vi "ScanFSM.vi"(0 "FSM X Task":refnum<k21>, 1 "FSM Y Task":refnum<k21>, 3 "Scan XY Map Progess Bar":refnum<vi>, 4 "XY Map Expected (s)":refnum<vi>, 5 "XY Map Elapsed (s)":refnum<vi>, 6 "XY Intensity Map":refnum<vi>, 7 "Scan X Readout (V)":refnum<vi>, 8 "CCD 1D Spectrum XY Map":refnum<vi>, 9 "LightField Automation out":refnum<class "LightField Automation.lvclass">, 10 "Params XY Map SubVI":T4, 11 "Scan Y Readout (V)":refnum<vi>, 12 "Scan XY Map Exp Params SubVI":T3, 13 "Stop XY Map":refnum<vi>, 14 "CCD 2D Image XY Map":refnum<vi>, 19 "LightField Automation error out":errorcluster) -> (16 "Data":i32[][](array[numeric]), 17 "LF Out":refnum<class "LightField Automation.lvclass">, 18 "LF Error Out":errorcluster)   [LabVIEW 2019]
uses:
  TypeDefs/AcqMode.ctl
  Light Field/lightfield-automation-labview/LightField Automation.lvclass
panel:
  out "size(s)":i32[](array[numeric])
  out "Numeric 2":i32
  out "Numeric":i32
  out "Number of points":dbl=121.0
  out "YMultiplier":dbl
  out "YOffset":dbl
  out "XMultiplier":dbl
  out "XOffset":dbl
  out "XYPos Indices Randomized":dbl[][](array[numeric])
  out "XYPos Indices":i32[][](array[numeric])
  out "Random index":i32[](array[numeric])=[4, 16, 17, 14, 92, 29, 8, 31, 42, 104, 84, 28, 85, 90, 13, 60, 120, 41, 111, 82, 69, 34, 7, 77, 47, 59, 65, 116, 24, 30, 113, 2, 63, 94, 106, 103, 71, 100, 22, 18, 32, 102, 19, 97, 44, 12, 0, 1, 109, 27, 88, 99, 51, 107, 76, 56, 81, 96, 72, 93, 74, 21, 5, 79, 9, 117, 38, 45, 25, 58, 105, 57, 40, 52, 23, 87, 89, 62, 26, 110, 37, 3, 101, 10, 54, 61, 83, 46, 86, 66, 68, 43, 108, 11, 67, 75, 6, 80, 49, 20, 112, 78, 115, 119, 95, 64, 73, 39, 15, 48, 55, 70, 50, 98, 91, 35, 53, 36, 118, 33, 114]
  out "X size":dbl=11.0
  out "Y size":dbl=11.0
  out "WL Calib":dbl[](array[numeric])
  out "CCD 1D Spectrum XY Map 2":cluster{dbl[], dbl[]}(graph)
  out "CCD ROI":T1(ring)
  out "Accumulations":dbl
  out "Acq Mode":T2=enum."Spectrum"
  out "KCube Shutter On?":bool
  out "A Time (ms)":dbl
  out "XY Intensity Map":dbl[][](graph)=[[3.904687043201515e-13, 6.684989195773002e-11, 3.649880430807626e-09, 6.355065252727497e-08, 3.5287820878809013e-07, 6.248749509463085e-07, 3.5287820878809013e-07, 6.355065252727497e-08, 3.649880430807626e-09, 6.684989195773002e-11, 3.904687043201515e-13], [6.684989195773002e-11, 1.1444983952148092e-08, 6.248749509463097e-07, 1.0880140221963334e-05, 6.041424029819161e-05, 0.0001069812317752422, 6.041424029819161e-05, 1.0880140221963334e-05, 6.248749509463097e-07, 1.1444983952148092e-08, 6.684989195773002e-11], [3.649880430807626e-09, 6.248749509463097e-07, 3.41170163237202e-05, 0.0005940355282204004, 0.003298505755939091, 0.005840977343195246, 0.003298505755939091, 0.0005940355282204004, 3.41170163237202e-05, 6.248749509463097e-07, 3.649880430807626e-09], [6.355065252727497e-08, 1.0880140221963334e-05, 0.0005940355282204004, 0.01034317319661825, 0.05743261926761737, 0.10170139230422684, 0.05743261926761737, 0.01034317319661825, 0.0005940355282204004, 1.0880140221963334e-05, 6.355065252727497e-08], [3.5287820878809013e-07, 6.041424029819161e-05, 0.003298505755939091, 0.05743261926761737, 0.31890655732397044, 0.5647181220077593, 0.31890655732397044, 0.05743261926761737, 0.003298505755939091, 6.041424029819161e-05, 3.5287820878809013e-07], [6.248749509463085e-07, 0.0001069812317752422, 0.005840977343195246, 0.10170139230422684, 0.5647181220077593, 1.0, 0.5647181220077593, 0.10170139230422684, 0.005840977343195246, 0.0001069812317752422, 6.248749509463085e-07], [3.5287820878809013e-07, 6.041424029819161e-05, 0.003298505755939091, 0.05743261926761737, 0.31890655732397044, 0.5647181220077593, 0.31890655732397044, 0.05743261926761737, 0.003298505755939091, 6.041424029819161e-05, 3.5287820878809013e-07], [6.355065252727497e-08, 1.0880140221963334e-05, 0.0005940355282204004, 0.01034317319661825, 0.05743261926761737, 0.10170139230422684, 0.05743261926761737, 0.01034317319661825, 0.0005940355282204004, 1.0880140221963334e-05, 6.355065252727497e-08], [3.649880430807626e-09, 6.248749509463097e-07, 3.41170163237202e-05, 0.0005940355282204004, 0.003298505755939091, 0.005840977343195246, 0.003298505755939091, 0.0005940355282204004, 3.41170163237202e-05, 6.248749509463097e-07, 3.649880430807626e-09], [6.684989195773002e-11, 1.1444983952148092e-08, 6.248749509463097e-07, 1.0880140221963334e-05, 6.041424029819161e-05, 0.0001069812317752422, 6.041424029819161e-05, 1.0880140221963334e-05, 6.248749509463097e-07, 1.1444983952148092e-08, 6.684989195773002e-11], [3.904687043201515e-13, 6.684989195773002e-11, 3.649880430807626e-09, 6.355065252727497e-08, 3.5287820878809013e-07, 6.248749509463085e-07, 3.5287820878809013e-07, 6.355065252727497e-08, 3.649880430807626e-09, 6.684989195773002e-11, 3.904687043201515e-13]]
  out "XY Map Expected (s)":dbl caption="Expected (s)"
  out "XY Map Elapsed (s)":dbl caption="Elapsed (s)"
  in  "DigNum Refnum":refnum<vi>
  out "XYPositions":dbl[][](array[numeric])=[[-0.09999999999999998, -0.3], [-0.09999999999999998, -0.19999999999999996], [-0.3, 0.4], [0.20000000000000007, -0.09999999999999998], [-0.5, -0.5], [0.0, 0.20000000000000007], [0.30000000000000004, 0.30000000000000004], [-0.3, -0.5], [-0.5, 0.10000000000000009], [0.0, 0.4], [0.20000000000000007, 0.10000000000000009], [0.30000000000000004, 0.0], [-0.09999999999999998, -0.4], [-0.4, -0.19999999999999996], [-0.5, -0.19999999999999996], [0.4, 0.4], [-0.5, -0.4], [-0.5, -0.3], [-0.19999999999999996, 0.10000000000000009], [-0.19999999999999996, 0.4], [0.4, -0.5], [0.0, 0.10000000000000009], [-0.19999999999999996, 0.0], [0.10000000000000009, 0.30000000000000004], [-0.3, 0.10000000000000009], [0.10000000000000009, -0.3], [0.20000000000000007, -0.4], [-0.09999999999999998, 0.0], [-0.4, -0.5], [-0.5, 0.0], [-0.3, 0.20000000000000007], [-0.5, 0.20000000000000007], [-0.19999999999999996, 0.20000000000000007], [0.5, 0.4], [-0.4, 0.5], [0.5, 0.0], [0.5, 0.20000000000000007], [0.20000000000000007, -0.19999999999999996], [0.10000000000000009, -0.5], [0.4, 0.30000000000000004], [0.10000000000000009, 0.10000000000000009], [-0.4, 0.10000000000000009], [-0.5, 0.30000000000000004], [0.30000000000000004, -0.19999999999999996], [-0.09999999999999998, -0.5], [0.10000000000000009, -0.4], [0.20000000000000007, 0.5], [-0.3, -0.3], [0.4, 0.5], [0.30000000000000004, 0.5], [0.5, -0.3], [-0.09999999999999998, 0.30000000000000004], [0.10000000000000009, 0.20000000000000007], [0.5, 0.10000000000000009], [0.20000000000000007, 0.20000000000000007], [0.5, -0.5], [0.0, -0.5], [0.10000000000000009, 0.0], [0.10000000000000009, -0.19999999999999996], [-0.3, -0.19999999999999996], [-0.4, -0.09999999999999998], [0.20000000000000007, 0.30000000000000004], [0.20000000000000007, -0.5], [-0.3, 0.5], [0.4, 0.10000000000000009], [-0.3, -0.09999999999999998], [0.30000000000000004, -0.4], [0.30000000000000004, 0.10000000000000009], [0.30000000000000004, -0.3], [-0.4, 0.4], [0.5, -0.4], [-0.19999999999999996, -0.19999999999999996], [0.0, -0.19999999999999996], [0.4, 0.20000000000000007], [0.0, 0.0], [0.30000000000000004, 0.20000000000000007], [-0.09999999999999998, 0.5], [-0.3, -0.4], [0.4, -0.3], [0.0, 0.30000000000000004], [0.30000000000000004, 0.4], [0.0, -0.4], [-0.4, 0.30000000000000004], [0.20000000000000007, 0.4], [-0.5, 0.5], [-0.4, -0.4], [0.30000000000000004, -0.5], [0.10000000000000009, 0.4], [-0.09999999999999998, 0.10000000000000009], [0.10000000000000009, 0.5], [-0.4, -0.3], [0.5, -0.09999999999999998], [-0.5, -0.09999999999999998], [0.0, -0.09999999999999998], [-0.19999999999999996, -0.5], [0.4, 0.0], [0.0, -0.3], [-0.19999999999999996, 0.5], [0.5, -0.19999999999999996], [-0.09999999999999998, 0.20000000000000007], [-0.19999999999999996, -0.09999999999999998], [0.20000000000000007, 0.0], [-0.19999999999999996, 0.30000000000000004], [-0.19999999999999996, -0.3], [-0.5, 0.4], [0.10000000000000009, -0.09999999999999998], [-0.19999999999999996, -0.4], [-0.09999999999999998, 0.4], [0.30000000000000004, -0.09999999999999998], [-0.09999999999999998, -0.09999999999999998], [0.20000000000000007, -0.3], [-0.4, 0.20000000000000007], [0.4, -0.4], [-0.3, 0.30000000000000004], [0.5, 0.5], [0.4, -0.19999999999999996], [-0.3, 0.0], [0.0, 0.5], [0.5, 0.30000000000000004], [0.4, -0.09999999999999998], [-0.4, 0.0]]
  out "Scan Y Res. (V)":dbl caption="Res. Y (V)"
  out "Scan Y Tot. Length":dbl caption="Y Length"
  out "Scan Y Center (V)":dbl caption="Y Center (V)"
  out "Scan Fast Axis":enum16{"Y", "X"}(ring)=enum."X" caption="Fast Axis"
  out "Scan X Res. (V)":dbl caption="Res. X (V)"
  out "Scan X Center (V)":dbl caption="X Center (V)"
  out "Scan X Tot. Length (V)":dbl caption="X Length (V)"
  out "Scanning Mode":T5(ring) caption="Mode"
  in  "Stop XY Map":bool
  out "Scan XY Map Progess Bar":u8(slide) scale=0.0..100.0
  out "CCD 2D Image XY Map":dbl[][](graph)
  out "Scan X Readout (V)":dbl caption="X Readout (V)" min=-10.0 max=10.0
  out "Scan Y Readout (V)":dbl caption="Y Readout (V)" min=-10.0 max=10.0
types:
  T1 = enum16{"Custom ROI", "Full sensor", "Binned full sensor"}
  T2 = typedef "AcqMode.ctl" = enum16{"Image", "Spectrum", "APD 1", "APD 2", "APD 1+2"}
  T3 = cluster{"Exposure Time (ms)":dbl, "Accumulations":dbl, "Excitation Wavelength (nm)":dbl, "Acq Mode":T2, "CCD ROI":enum16{"Custom ROI", "Full sensor", "Binned full sensor"}, "KCube Shutter On?":bool}
  T4 = cluster{"Scan Fast Axis":enum16{"Y", "X"}, "Scanning Mode":enum16{"Default", "Snail", "Random", "Snake", "Line"}, "Scan X Center (V)":dbl, "Scan X Res. (V)":dbl, "Scan X Tot. Length (V)":dbl, "Scan Y Center (V)":dbl, "Scan Y Res. (V)":dbl, "Scan Y Tot. Length":dbl}
  T5 = enum16{"Default", "Snail", "Random", "Snake", "Line"}
  T6 = enum16{"Image", "Spectrum", "APD 1", "APD 2", "APD 1+2"}
  T7 = enum16{"Contrast", "Spectre", "Polarisation", "Time Trace", "XY Intensity Map"}
  T8 = cluster{"Image":dbl[][][], "Frame Size":cluster{"F":i32, "Y":i32, "X":i32}}[]
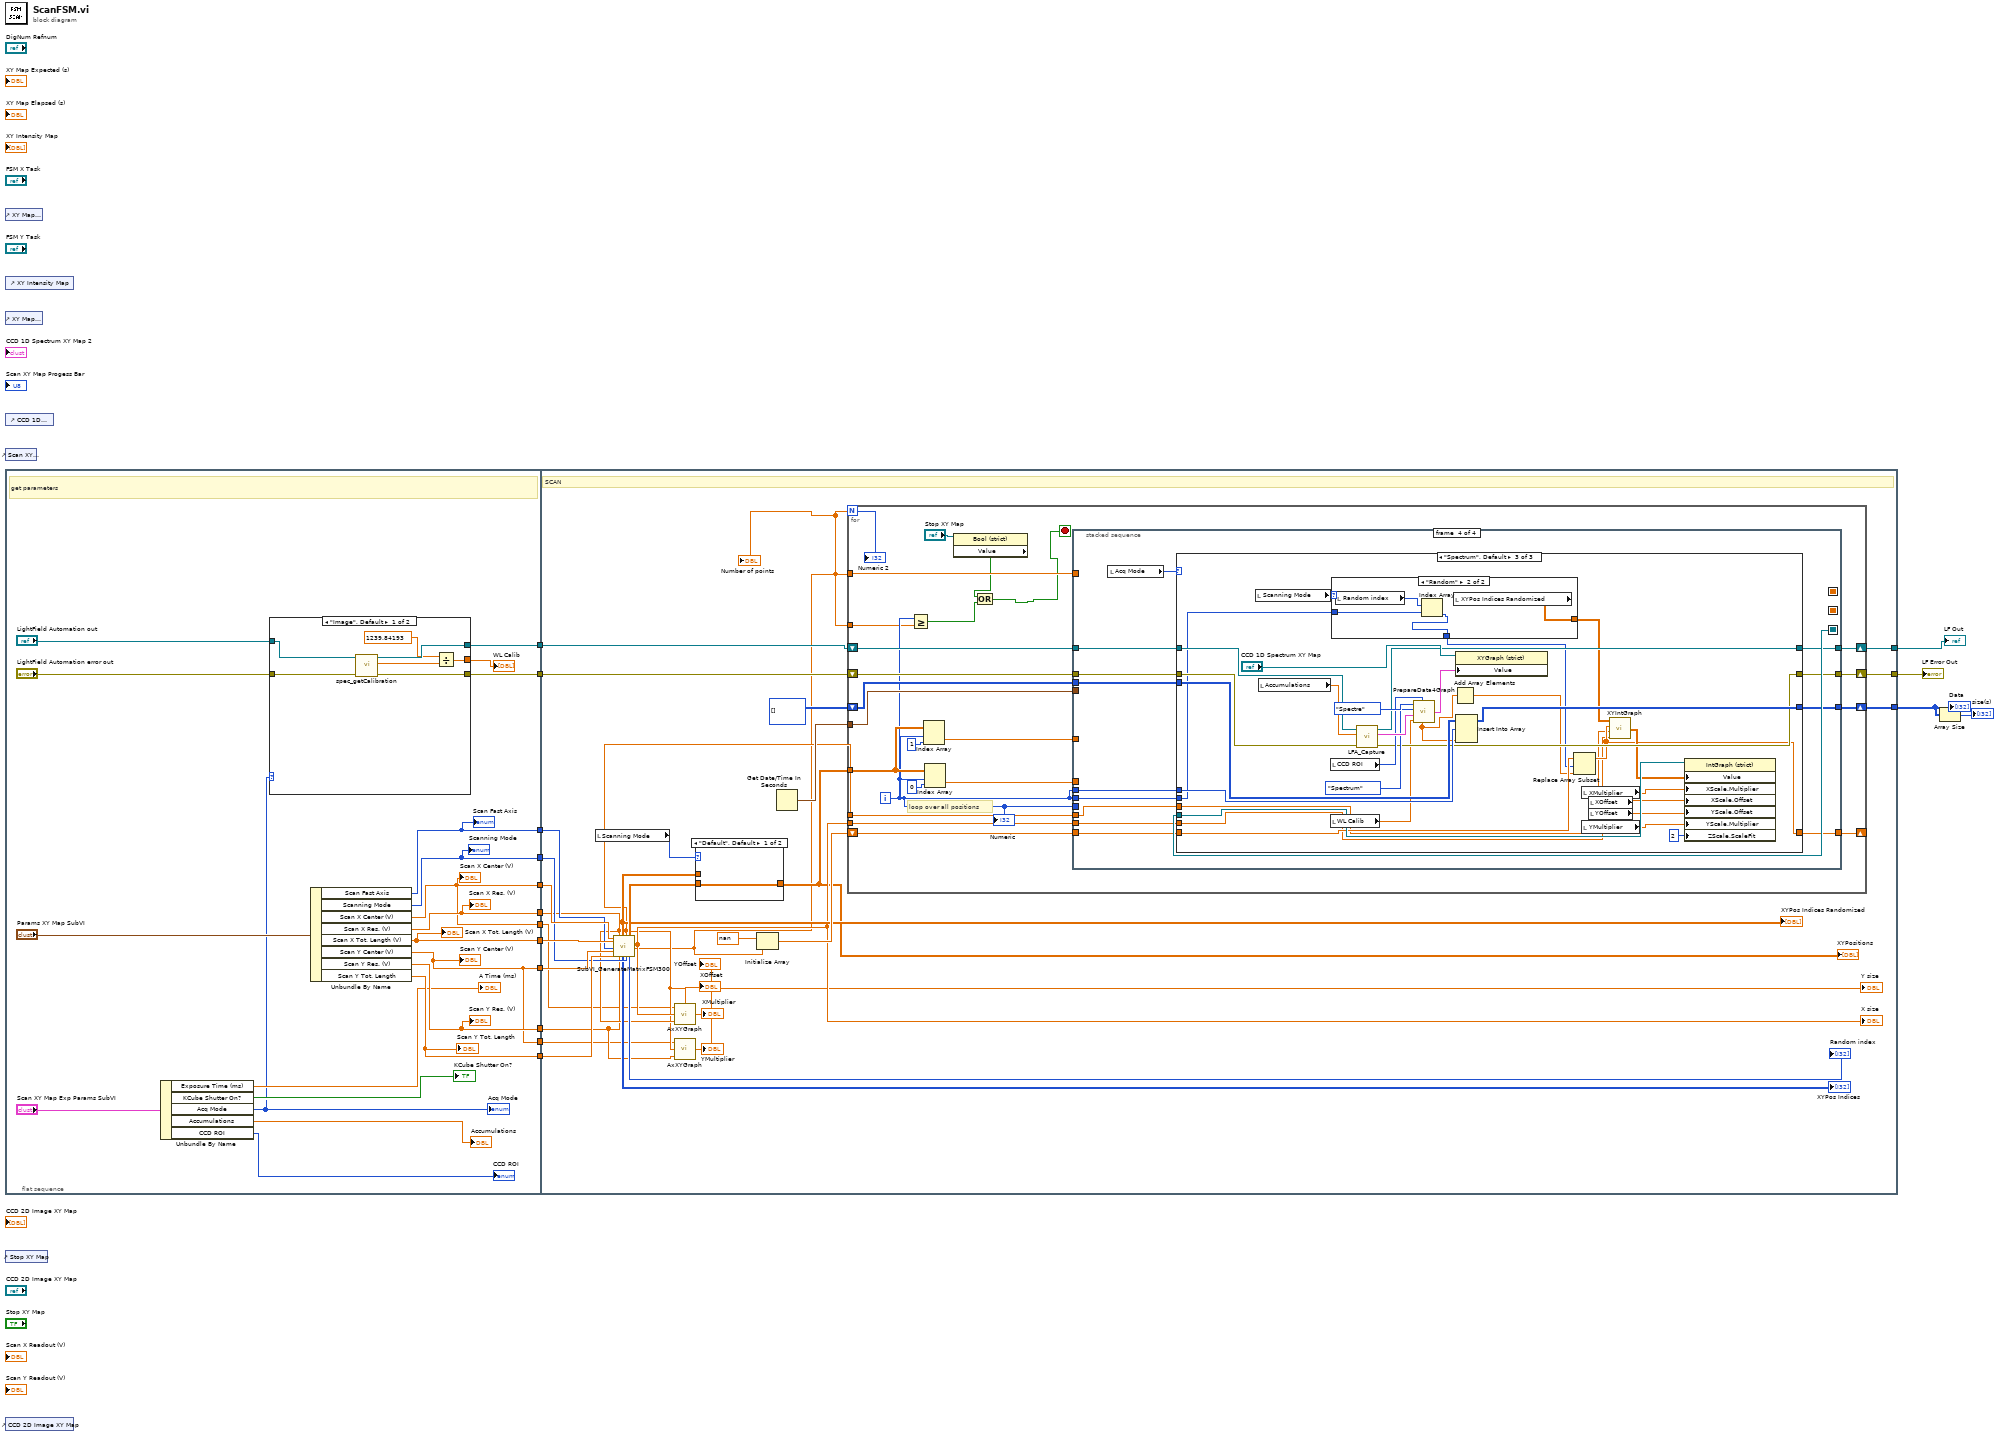
[diagram p0: block diagram]
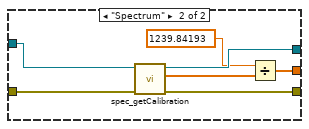
[diagram p2: hidden frame]
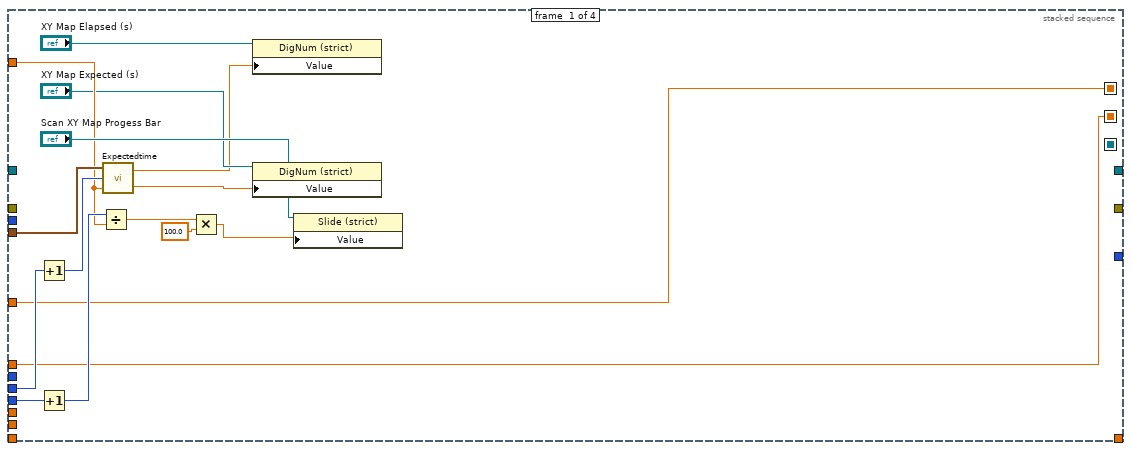
[diagram p4: hidden frame]
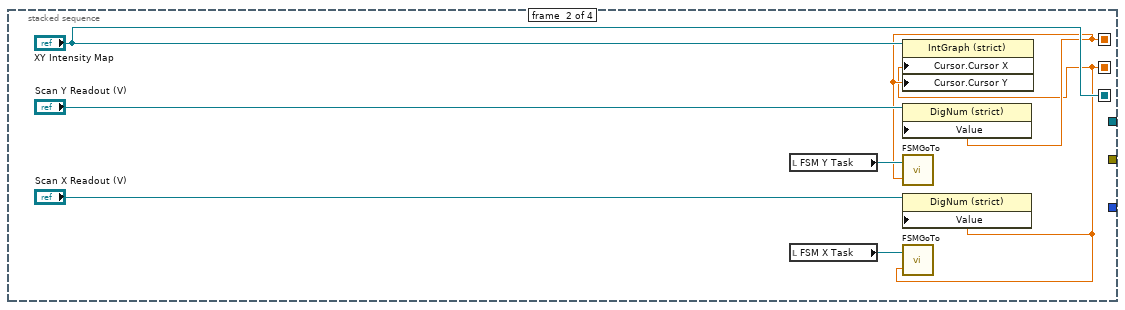
[diagram p5: hidden frame]
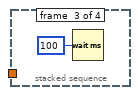
[diagram p6: hidden frame]
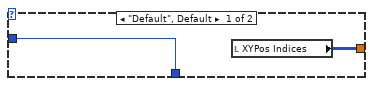
[diagram p9: hidden frame]
diagram:
  n1 = control-ref of="XY Map Expected (s)"() -> ()  [unwired: 1 out]
  n2 = control-ref of="XY Intensity Map"() -> ()  [unwired: 1 out]
  n3 = control-ref of="XY Map Elapsed (s)"() -> ()  [unwired: 1 out]
  n4 = control-ref of="CCD 1D Spectrum XY Map"() -> ()  [unwired: 1 out]
  n5 = control-ref of="Scan XY Map Progess Bar"() -> ()  [unwired: 1 out]
  n6 = flat-sequence {
    tunnel: [w35] -> w16
    tunnel: [w18] -> w15
    tunnel: [w34] -> w14
    tunnel: [w33] -> w13
    tunnel: [w17] -> w12
    tunnel: [w32] -> w11
    tunnel: [w31] -> w10
    tunnel: [w30] -> w9
    tunnel: [w21] -> w6
    tunnel: [w20] -> w5
    tunnel: [w18] -> w4
    tunnel: [w17] -> w3
    tunnel: w16 -> [w62]
    tunnel: w15 -> [w81]
    tunnel: w14 -> [w80]
    tunnel: w13 -> [w79]
    tunnel: w12 -> [w78]
    tunnel: w11 -> [w77]
    tunnel: w10 -> [w58]
    tunnel: w9 -> [w76]
    tunnel: [w74] -> w2
    tunnel: [w73] -> w8
    tunnel: [w72] -> w7
    tunnel: w6 -> [w71]
    tunnel: w5 -> [w70]
    tunnel: w4 -> [w55]
    tunnel: w3 -> [w54]
    frame #0 {
      # "get parameters"
      n7 = Unbundle By Name("Scan XY Map Exp Params SubVI") -> ("Exposure Time (ms)"=→"A Time (ms)":dbl, "KCube Shutter On?"=→"KCube Shutter On?":bool, "Acq Mode"=w24:T2, "Accumulations"=→"Accumulations":dbl, "CCD ROI"=→"CCD ROI":T1)
      "Acq Mode" <- w24
      n8 = case shown="\"Image\", Default" w24 {
        tunnel: "LightField Automation out" -> [w43 w50]
        tunnel: "LightField Automation error out" -> [w42 w49]
        tunnel: [w41 w48] -> w21
        tunnel: [w40 w47] -> w20
        tunnel: [w37 w44] -> w19
        frame "Image", Default {
          n9 = call "spec_getCalibration.vi"("error in (no error)"=w42, "LightField Automation in"=w43) -> ("error out"=w40:errorcluster, "ColumnCalibration"=w38:dbl[], "LightField Automation out"=w41:refnum<class "LightField Automation.lvclass">)  [unwired: 7 in]
          n10 = Divide(x=1239.84193, y=w38) -> (x/y=w37:dbl[])
        }
        frame "Spectrum" {
          n11 = call "spec_getCalibration.vi"("error in (no error)"=w49, "LightField Automation in"=w50) -> ("error out"=w47:errorcluster, "ColumnCalibration"=w45:dbl[], "LightField Automation out"=w48:refnum<class "LightField Automation.lvclass">)  [unwired: 7 in]
          n12 = Divide(x=1239.84193, y=w45) -> (x/y=w44:dbl[])
        }
      }
      "WL Calib" <- w19
      n13 = Unbundle By Name("Params XY Map SubVI") -> ("Scan Fast Axis"=w33:enum16{"Y", "X"}, "Scanning Mode"=w30:T5, "Scan X Center (V)"=w18:dbl, "Scan X Res. (V)"=w35:dbl, "Scan X Tot. Length (V)"=w34:dbl, "Scan Y Center (V)"=w17:dbl, "Scan Y Res. (V)"=w31:dbl, "Scan Y Tot. Length"=w32:dbl)
      "Scan X Tot. Length (V)" <- w34
      "Scan X Res. (V)" <- w35
      "Scan Y Center (V)" <- w17
      "Scan Y Tot. Length" <- w32
      "Scan Y Res. (V)" <- w31
      "Scanning Mode" <- w30
      "Scan X Center (V)" <- w18
      "Scan Fast Axis" <- w33
    }
    frame #1 {
      # "SCAN"
      n14 = local read "Scanning Mode"() -> (w66:T5)
      n15 = call "SubVI_GenerateMatrixFSM300.vi"("X center (Volt)"=w81, "Total Length X (Volt)"=w80, "''fast mooving'' axis"=w79, "Y center (Volt)"=w78, "Total Length Y (Volt)"=w77, "Resolution X (Volt)"=w62, "Resolution Y (Volt)"=w58, "Scan mode"=w76) -> ("XYPos Indices Randomized"=w64:dbl[][], "XYPos Indices"=→"XYPos Indices":i32[][], "Y size"=w59:dbl, "XYPositions"=w65:dbl[][], "Random index"=→"Random index":i32[], "X size"=w63:dbl, "Number of points"=w52:dbl)  [unwired: 1 in, 4 out]
      "Y size" <- w59
      "X size" <- w63
      "XYPos Indices Randomized" <- w64
      "Number of points" <- w52
      n16 = call "AxXYGraph.vi"("dx"=w62, "N"=w63, "x0"=w55) -> ("Multiplier"=→"XMultiplier":dbl, "Offset"=→"XOffset":dbl)
      n17 = call "AxXYGraph.vi"("dx"=w58, "N"=w59, "x0"=w54) -> ("Multiplier"=→"YMultiplier":dbl, "Offset"=→"YOffset":dbl)
      n18 = case shown="\"Default\", Default" w66 {
        tunnel: w65 -> [w83 w84]
        tunnel: [w83 w84] -> w53
        tunnel: w64 -> [_ _]
        frame "Default", Default {
        }
        frame "Random" {
        }
      }
      "XYPositions" <- w53
      n19 = Initialize Array(nan, w52) -> (w68:dbl[])
      n20 = Get Date/Time In Seconds() -> (seconds since 1Jan1904=w82:timestamp)
      n21 = for {
        N: w52 -> [w90]
        tunnel: w53 -> [w108]
        tunnel: w82 -> [w102]
        shift-right: [w100] -> w74
        shift-left: i32[][] [] -> [w101]
        shift-right: [w99] -> w73
        shift-left: w71 -> [w98]
        shift-right: [w96] -> w72
        shift-left: w70 -> [w97]
        shift-right: [w94] -> _
        shift-left: w68 -> [w95]
        tunnel: w63 -> [w93]
        tunnel: w59 -> [w92]
        tunnel: w52 -> [w91]
        tunnel: w52 -> [w88]
        i -> [w89]
        stop <- w85 stop-if-true
        # "loop over all positions"
        n22 = Greater Or Equal?(x=w89, y=w88) -> (x >= y?=w87:bool)
        n23 = Index Array(array=w108, index (row)=w89, index (col)=1 ("index")) -> (element=w105:dbl)
        n24 = Index Array(array=w108, index (row)=w89, index (col)=0 ("index")) -> (element=w104:dbl)
        n25 = property class="Bool (strict)"(reference="Stop XY Map") -> ("Value"=w86:bool)  [unwired: 1 in, 2 out]
        n26 = Or(x=w86, y=w87) -> (x .or. y?=w85:bool)
        n27 = stacked-sequence {
          seq-local: [w111 _ _ _] -> [_ w126 _ _]
          seq-local: [w110 _ _ _] -> [_ w125 _ _]
          seq-local: [_ "XY Intensity Map" _ _] -> [_ _ _ w145]
          tunnel: w105 -> [w111 _ _ _]
          tunnel: w104 -> [w110 _ _ _]
          tunnel: w89 -> [w124 _ _ _]
          tunnel: w91 -> [w116 _ _ _]
          tunnel: w102 -> [w119 _ _ _]
          tunnel: w89 -> [w118 _ _ w136]
          tunnel: w101 -> [_ _ _ w144]
          tunnel: w89 -> [_ _ _ w143]
          tunnel: [_ _ _ w142] -> w100
          tunnel: [_ _ _ w141] -> w99
          tunnel: w98 -> [_ _ _ w140]
          tunnel: w97 -> [_ _ _ w139]
          tunnel: [_ _ _ w138] -> w96
          tunnel: w95 -> [_ _ _ w137]
          tunnel: [_ _ _ w135] -> w94
          tunnel: w93 -> [_ _ _ w134]
          tunnel: w92 -> [_ _ _ w133]
          frame #0 {
            n28 = Increment(x=w118) -> (x+1=w117:i32)
            n29 = Increment(x=w124) -> (x+1=w123:i32)
            n30 = Divide(x=w123, y=w116) -> (x/y=w121:dbl)
            n31 = call "Expectedtime.vi"("N"=w116, "I"=w117, "Reference time"=w119) -> ("Expected time"=w114:dbl, "Elapsed time"=w112:dbl)
            n32 = Multiply(x=w121, y=100.0 ("x/y")) -> (x*y=w109:dbl)
            n33 = property class="DigNum (strict)"(reference="XY Map Elapsed (s)", "Value"=w112) -> ()  [unwired: 1 in, 2 out]
            n34 = property class="DigNum (strict)"(reference="XY Map Expected (s)", "Value"=w114) -> ()  [unwired: 1 in, 2 out]
            n35 = property class="Slide (strict)"(reference="Scan XY Map Progess Bar", "Value"=w109) -> ()  [unwired: 1 in, 2 out]
          }
          frame #1 {
            n36 = local read "FSM Y Task"() -> (w131:refnum<k21>)
            n37 = local read "FSM X Task"() -> (w130:refnum<k21>)
            n38 = property class="IntGraph (strict)"(reference="XY Intensity Map", "Cursor.Cursor X"=w125, "Cursor.Cursor Y"=w126) -> ()  [unwired: 1 in, 2 out]
            n39 = property class="DigNum (strict)"(reference="Scan Y Readout (V)", "Value"=w126) -> ()  [unwired: 1 in, 2 out]
            n40 = call "FSMGoTo.vi"("Target Value (V)"=w126, "FSM Task"=w131) -> ()  [unwired: 1 out]
            n41 = property class="DigNum (strict)"(reference="Scan X Readout (V)", "Value"=w125) -> ()  [unwired: 1 in, 2 out]
            n42 = call "FSMGoTo.vi"("Target Value (V)"=w125, "FSM Task"=w130) -> ()  [unwired: 1 out]
          }
          frame #2 {
            n43 = Wait (ms)(milliseconds to wait=u32 100) -> ()  [unwired: 1 out]
          }
          frame #3 {
            n44 = local read "Acq Mode"() -> (w146:T2)
            n45 = case shown="\"Spectrum\", Default" w146 {
              tunnel: w140 -> [w149 w153 w186]
              tunnel: w139 -> [w148 w152 w185]
              tunnel: w145 -> [_ _ w179]
              tunnel: w144 -> [w150 w154 w176]
              tunnel: w143 -> [_ _ w175]
              tunnel: [w150 w154 w174] -> w142
              tunnel: [w149 w153 w173] -> w141
              tunnel: [w148 w152 w172] -> w138
              tunnel: w137 -> [w147 w151 w169]
              tunnel: w136 -> [_ _ w157]
              tunnel: [w147 w151 w166] -> w135
              tunnel: w134 -> [_ _ w158]
              tunnel: w133 -> [_ _ w165]
              frame "Image" {
              }
              frame "APD 1" {
              }
              frame "Spectrum", Default {
                n46 = local read "Scanning Mode"() -> (w164:T5)
                n47 = local read "Accumulations"() -> (w184:dbl)
                n48 = local read "CCD ROI"() -> (w180:T1)
                n49 = local read "WL Calib"() -> (w171:dbl[])
                n50 = case shown="\"Random\"" w164 {
                  tunnel: [w188 w192] -> w163
                  tunnel: w157 -> [w187 w190]
                  tunnel: [w187 w189] -> w156
                  frame "Default", Default {
                    n51 = local read "XYPos Indices"() -> (w188:i32[][])
                  }
                  frame "Random" {
                    n52 = local read "Random index"() -> (w191:i32[])
                    n53 = Index Array(array=w191, index=w190) -> (element=w189:i32)
                    n54 = local read "XYPos Indices Randomized"() -> (w192:dbl[][])
                  }
                }
                n55 = call "LFA_Capture.vi"("error in (no error)"=w185, "Frames"=w184, "LightField Automation in"=w186) -> ("error out"=w172:errorcluster, "Data"=w183:T8, "LightField Automation out"=w173:refnum<class "LightField Automation.lvclass">)  [unwired: 6 in]
                n56 = call "PrepareData4Graph.vi"("Wavelength nm"=w171, "DataLF"=w183, "CCD ROI"=w180, "AcqMode"=T6."Spectrum", "Data type"=T7."Spectre") -> ("Spectrum"=w177:cluster{"Array 2":dbl[], "Array":dbl[]}, "PLInt out"=w168:dbl[])  [unwired: 2 in, 2 out]
                n57 = Add Array Elements(numeric array=w168) -> (sum=w167:dbl)
                n58 = property class="XYGraph (strict)"(reference="CCD 1D Spectrum XY Map", "Value"=w177) -> ()  [unwired: 1 in, 2 out]
                n59 = Insert Into Array(array=w176, index (row)=w175, new element=w168) -> (w174:i32[][])  [unwired: 1 in]
                n60 = Replace Array Subset(array=w169, new element=w167, index=w156) -> (w166:dbl[])
                n61 = local read "XMultiplier"() -> (w162:dbl)
                n62 = local read "YMultiplier"() -> (w159:dbl)
                n63 = local read "XOffset"() -> (w161:dbl)
                n64 = local read "YOffset"() -> (w160:dbl)
                n65 = call "XYIntGraph.vi"("Columns"=w158, "Rows"=w165, "Z Intensity"=w166, "XY Pos"=w163) -> ("Intensity Graph"=w170:dbl[][])
                n66 = property class="IntGraph (strict)"(reference=w179, "Value"=w170, "XScale.Multiplier"=w162, "XScale.Offset"=w161, "YScale.Offset"=w160, "YScale.Multiplier"=w159, "ZScale.ScaleFit"=u8 2 ("Z Scale.Scale Fit")) -> ()  [unwired: 1 in, 2 out]
              }
            }
          }
        }
        "Numeric" <- w89
        "Numeric 2" <- w90
      }
    }
  }
  n67 = control-ref of="Stop XY Map"() -> ()  [unwired: 1 out]
  n68 = control-ref of="CCD 2D Image XY Map"() -> ()  [unwired: 1 out]
  n69 = Array Size(array=w2) -> (size(s)=→"size(s)":i32[])
  "Data" <- w2
  "LF Out" <- w8
  "LF Error Out" <- w7
